vi "Repack Pixels_FIFO to Pixel Bus U8x8.vi"(8 "Last \npacket length":u8, 9 "Last valid \npacket - Image":bool, 10 "Last valid \npacket - Row":bool, 11 "Source Image FIFO":refnum<k21>) -> (1 "Read/No Read":bool, 2 "DV Out":bool, 3 "Pixel Bus Out":T1={"Pixel Data"=[0, 0, 0, 0, 0, 0, 0, 0], "DV"=[FALSE, FALSE, FALSE, FALSE, FALSE, FALSE, FALSE, FALSE], "EOL"=FALSE, "EOI"=FALSE, "Data Type"=enum."U8 x 8"})   [LabVIEW 2017, in "NI_VDM_FPGA_Basics.lvlib"]
uses:
  <vilib>/visionFPGA/NI_VDM_FPGA_Basics.lvlib
  <vilib>/rvi/DataTransferAndStorage/Container/XNode/niFpgaContainer.xnode
  <vilib>/visionFPGA/Controls/IMAQ FPGA Pixel Bus u8x8.ctl
  <vilib>/rvi/FIFO/Fifo_Resource/niFpgaFifoEmulationRefInMultiElement.vi
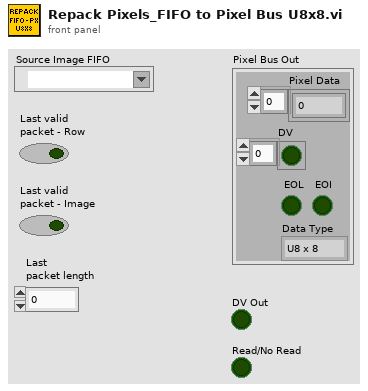
[diagram p1: front panel]
types:
  T1 = typedef "IMAQ FPGA Pixel Bus u8x8.ctl" = cluster{"Pixel Data":u8[], "DV":bool[], "EOL":bool, "EOI":bool, "Data Type":enum16{"U8 x 8"}}
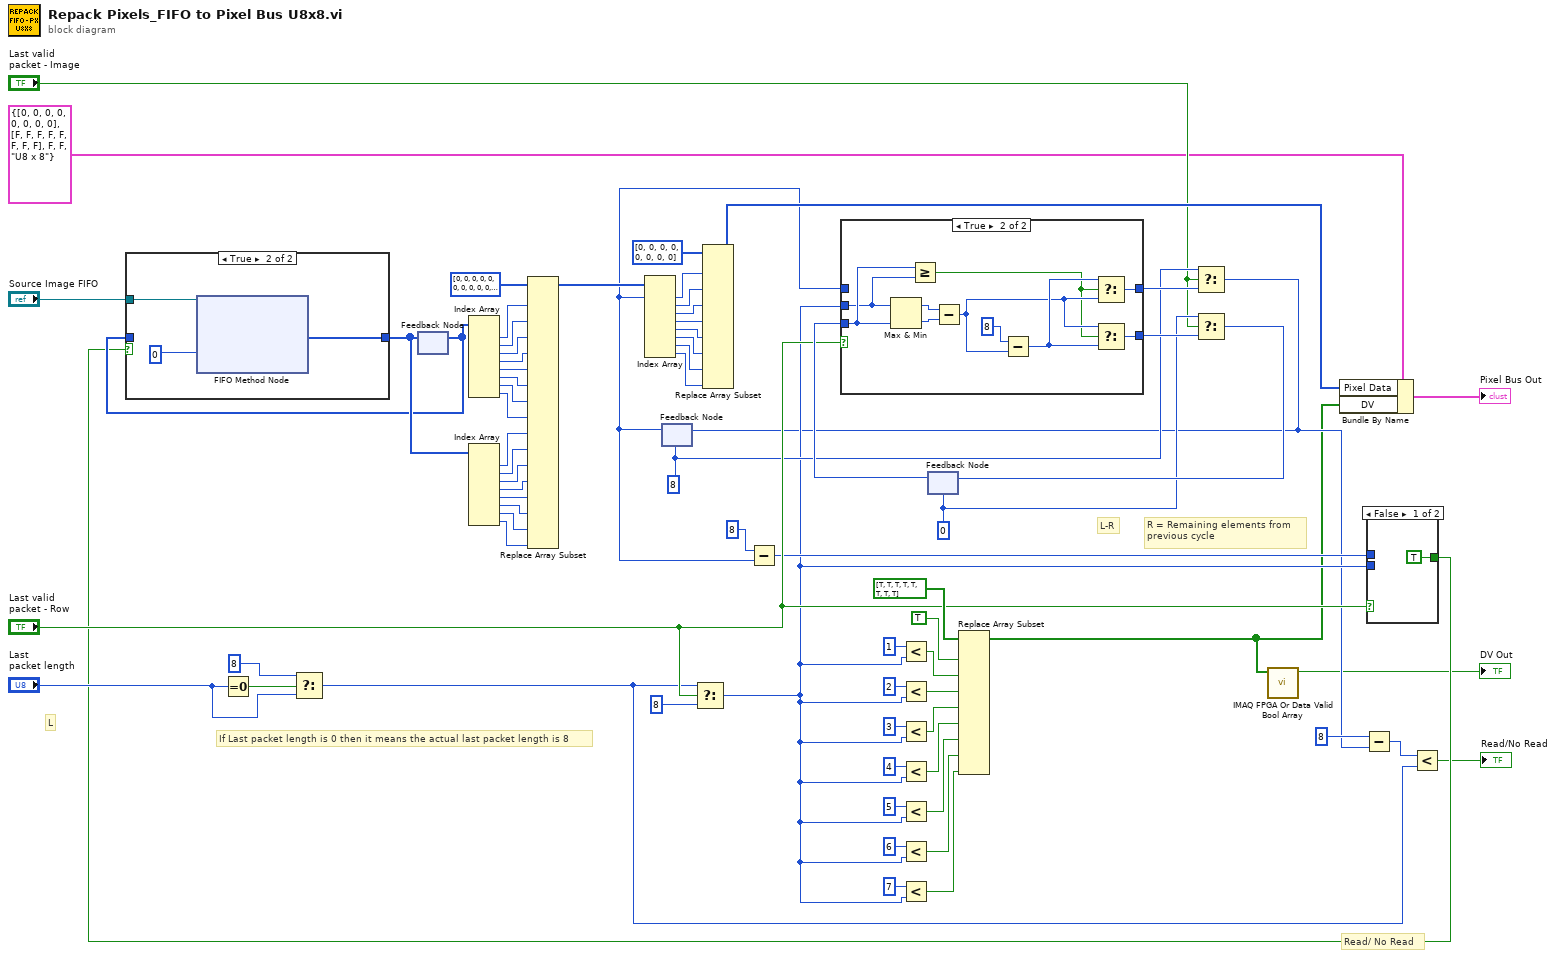
[diagram p0: block diagram]
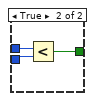
[diagram p3: hidden frame]
diagram:
  w15 = u8 0
  w16 = u8 8
  # "L"
  # "L-R"
  # "If Last packet length is 0 then it means the actual last packet length is 8"
  # "Read/ No Read"
  # "R = Remaining elements from\nprevious cycle"
  n1 = Equal To 0?(x="Last \npacket length") -> (x = 0?=w36:bool)
  n2 = Select(t=u8 8, s=w36, f="Last \npacket length") -> (s? t:f=w5:u8)
  n3 = feedback #1() -> (w21:u8[])  [unwired: 1 in]
  n4 = Index Array(array=w21) -> (element #1=w55:u8, element #2=w54:u8, element #3=w53:u8, element #4=w52:u8, element #5=w51:u8, element #6=w50:u8, element #7=w49:u8, element #8=w48:u8)  [unwired: 8 in]
  n5 = feedback #2(w16) -> (w13:u8)
  n6 = Select(t=w5, s="Last valid \npacket - Row", f=u8 8) -> (s? t:f=w10:u8)
  n7 = Subtract(x=u8 8, y=w13) -> (x-y=w11:u8)
  n8 = Less?(x=u8 1, y=w10) -> (x < y?=w62:bool)
  n9 = Less?(x=u8 2, y=w10) -> (x < y?=w61:bool)
  n10 = Less?(x=u8 3, y=w10) -> (x < y?=w60:bool)
  n11 = Less?(x=u8 4, y=w10) -> (x < y?=w59:bool)
  n12 = Less?(x=u8 5, y=w10) -> (x < y?=w58:bool)
  n13 = Less?(x=u8 6, y=w10) -> (x < y?=w57:bool)
  n14 = Less?(x=u8 7, y=w10) -> (x < y?=w56:bool)
  n15 = feedback #3(w15) -> (w24:u8)
  n16 = case shown="True" "Last valid \npacket - Row" {
    tunnel: w24 -> [w74 w85]
    tunnel: w10 -> [_ w84]
    tunnel: [w75 w83] -> w18
    tunnel: [w74 w82] -> w17
    tunnel: w13 -> [w75 _]
    frame False {
    }
    frame True {
      n17 = Max & Min(x=w84, y=w85) -> (max(x,y)=w79:u8, min(x,y)=w78:u8)
      n18 = Greater Or Equal?(x=w85, y=w84) -> (x >= y?=w76:bool)
      n19 = Subtract(x=w79, y=w78) -> (x-y=w80:u8)
      n20 = Subtract(x=u8 8, y=w80) -> (x-y=w81:u8)
      n21 = Select(t=w81, s=w76, f=w80) -> (s? t:f=w83:u8)
      n22 = Select(t=w80, s=w76, f=w81) -> (s? t:f=w82:u8)
    }
  }
  n23 = Replace Array Subset(array=bool[] [TRUE, TRUE, TRUE, TRUE, TRUE, TRUE, TRUE, TRUE], new element #1=TRUE ("new element/subarray"), new element #2=w62, new element #3=w61, new element #4=w60, new element #5=w59, new element #6=w58, new element #7=w57, new element #8=w56) -> (w2:bool[])  [unwired: 8 in]
  n24 = Select(t=w16, s="Last valid \npacket - Image", f=w18) -> (s? t:f=w8:u8)
  n25 = feedback-in #2(w8) -> ()
  n26 = Select(t=w15, s="Last valid \npacket - Image", f=w17) -> (s? t:f=w19:u8)
  n27 = feedback-in #3(w19) -> ()
  n28 = call <vilib>:"IMAQ FPGA Or Data Valid Bool Array.vi"("DV Array In"=w2) -> ("DV Out"=→"DV Out":bool)  [unwired: 10 in]
  n29 = Subtract(x=u8 8, y=w8) -> (x-y=w7:u8)
  n30 = case shown="False" "Last valid \npacket - Row" {
    tunnel: w10 -> [_ w88]
    tunnel: w11 -> [_ w89]
    tunnel: [TRUE w87] -> w12
    frame False {
    }
    frame True {
      n31 = Less?(x=w89, y=w88) -> (x < y?=w87:bool)
    }
  }
  n32 = case shown="True" w12 {
    tunnel: "Source Image FIFO" -> [_ w93]
    tunnel: [w90 w91] -> w47
    tunnel: w21 -> [w90 _]
    frame False {
    }
    frame True {
      n33 = xnode ("FIFO Method Node")("Timeout"=0, "FIFO In"=w93) -> ("Element"=w91:u8[])  [unwired: 2 out]
    }
  }
  n34 = feedback-in #1(w47) -> ()
  n35 = Index Array(array=w47) -> (element #1=w46:u8, element #2=w45:u8, element #3=w44:u8, element #4=w43:u8, element #5=w42:u8, element #6=w41:u8, element #7=w40:u8, element #8=w39:u8)  [unwired: 8 in]
  n36 = Replace Array Subset(array=u8[] [0, 0, 0, 0, 0, 0, 0, 0, 0, 0, 0, 0, 0, 0, 0, 0], new element #1=w55, new element #2=w54, new element #3=w53, new element #4=w52, new element #5=w51, new element #6=w50, new element #7=w49, new element #8=w48, new element #9=w46, new element #10=w45, new element #11=w44, new element #12=w43, new element #13=w42, new element #14=w41, new element #15=w40, new element #16=w39) -> (w23:u8[])  [unwired: 16 in]
  n37 = Index Array(array=w23, index #1=w13) -> (element #1=w33:u8, element #2=w32:u8, element #3=w31:u8, element #4=w30:u8, element #5=w29:u8, element #6=w28:u8, element #7=w27:u8, element #8=w26:u8)  [unwired: 7 in]
  n38 = Replace Array Subset(array=u8[] [0, 0, 0, 0, 0, 0, 0, 0], new element #1=w33, new element #2=w32, new element #3=w31, new element #4=w30, new element #5=w29, new element #6=w28, new element #7=w27, new element #8=w26) -> (w22:u8[])  [unwired: 8 in]
  n39 = Bundle By Name(cluster=T1 {"Pixel Data"=[0, 0, 0, 0, 0, 0, 0, 0], "DV"=[FALSE, FALSE, FALSE, FALSE, FALSE, FALSE, FALSE, FALSE], "EOL"=FALSE, "EOI"=FALSE, "Data Type"=enum."U8 x 8"} ("Pixel Bus Out"), "Pixel Data"=w22, "DV"=w2) -> (→"Pixel Bus Out":T1)
  n40 = Less?(x=w7, y=w5) -> (x < y?=→"Read/No Read":bool)
